vi "add_default_value_on_label.vi"(8 "error in (no error)":errorcluster, 11 "VI Ref In":refnum<vi>) -> (0 "error out":errorcluster, 3 "VI Ref Out":refnum<vi>)   [LabVIEW 2018]
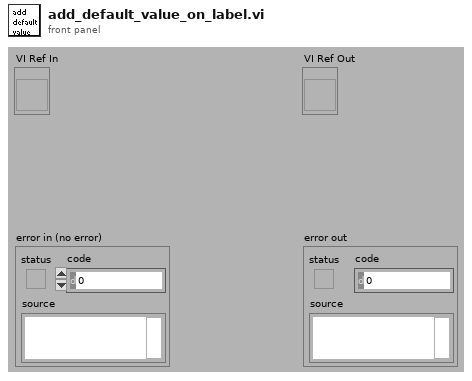
[diagram p1: front panel]
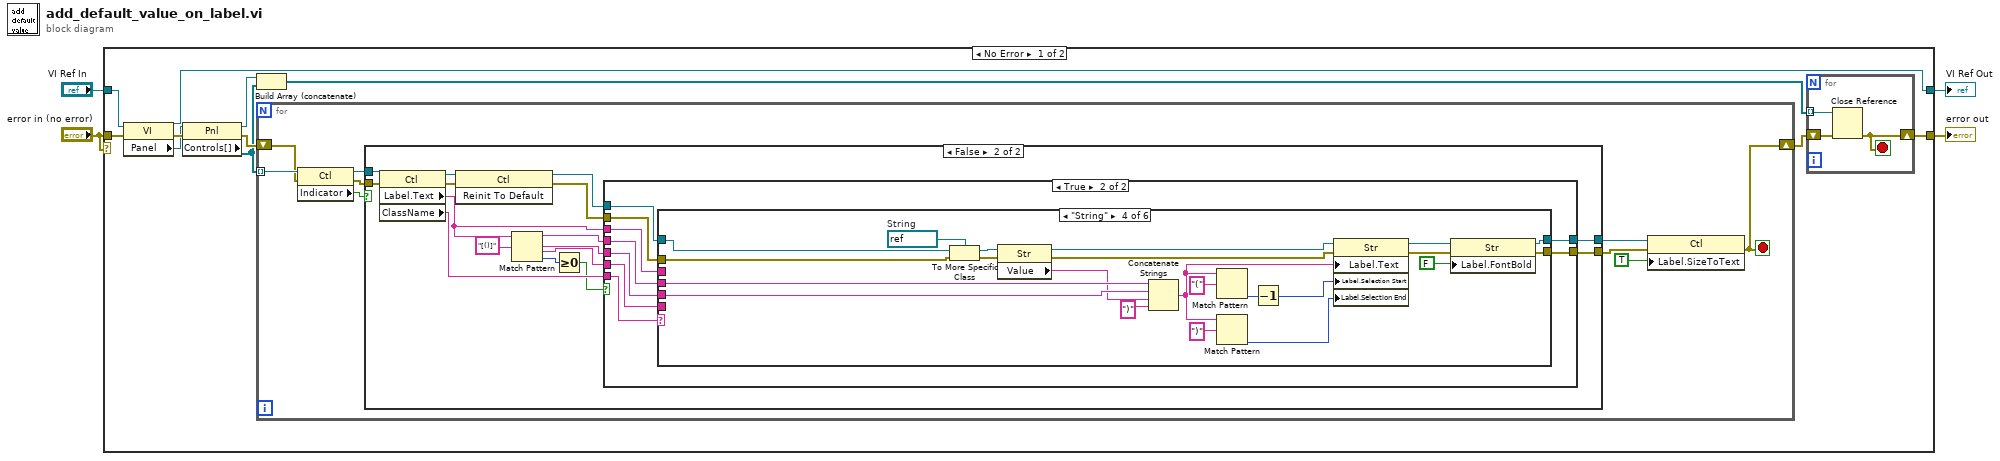
[diagram p0: block diagram]
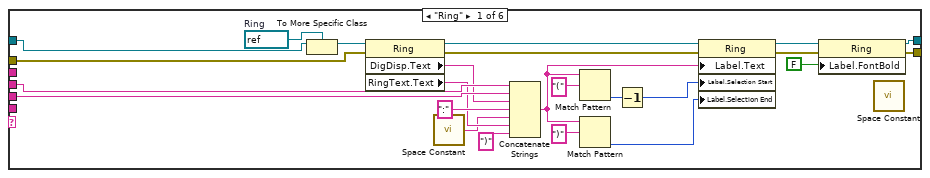
[diagram p4: hidden frame]
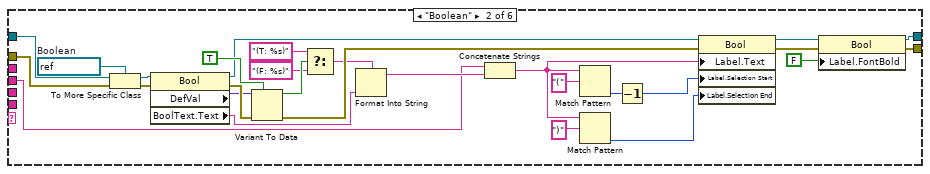
[diagram p5: hidden frame]
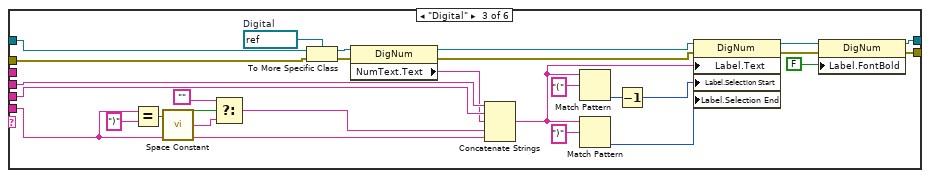
[diagram p6: hidden frame]
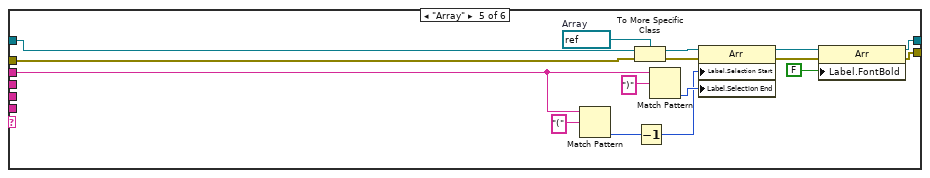
[diagram p7: hidden frame]
diagram:
  n1 = case shown="No Error" "error in (no error)" {
    tunnel: [w9 w177] -> w4
    tunnel: "VI Ref In" -> [w6 w177]
    tunnel: "error in (no error)" -> [w8 w176]
    tunnel: [w7 w176] -> w3
    frame No Error {
      n2 = property class="VI"(reference=w6, error in=w8) -> (reference out=w9:refnum<vi>, error out=w15:errorcluster, "Panel"=w5:refnum<vi>)
      n3 = property class="Pnl"(reference=w5, error in=w15) -> (reference out=w13:refnum<vi>, error out=w14:errorcluster, "Controls[]"=w12:refnum<vi>[])
      n4 = Build Array (concatenate)(w13, w12) -> (w11:refnum<vi>[])
      n5 = for {
        tunnel: w12 -> [w25] mode=indexing
        shift-right: [w19] -> w10
        shift-left: w14 -> [w22]
        stop <- w19 stop-if-true
        n6 = property class="Ctl"(reference=w25, error in=w22) -> (reference out=w23:refnum<vi>, error out=w21:errorcluster, "Indicator"=w24:bool)
        n7 = case shown="False" w24 {
          tunnel: w21 -> [w28 w45]
          tunnel: [w28 w42] -> w20
          tunnel: [w29 w41] -> w27
          tunnel: w23 -> [w29 w40]
          frame True {
          }
          frame False {
            n8 = property class="Ctl"(reference=w40, error in=w45) -> (reference out=w39:refnum<vi>, error out=w38:errorcluster, "Label.Text"=w30:string, "ClassName"=w44:string)
            n9 = invoke class="Ctl" method="Reinit To Default"(reference=w39, error in=w38) -> (reference out=w36:refnum<vi>, error out=w37:errorcluster)  [unwired: 1 in, 1 out]
            n10 = Match Pattern(string=w30, regular expression="[()]") -> (before substring=w33:string, match substring=w32:string, after substring=w31:string, offset past match=w35:i32)  [unwired: 1 out]
            n11 = Greater Or Equal To 0?(x=w35) -> (x >= 0?=w34:bool)
            n12 = case shown="True" w34 {
              tunnel: w37 -> [w47 w56]
              tunnel: w44 -> [_ w54]
              tunnel: w36 -> [w46 w55]
              tunnel: [w47 w53] -> w42
              tunnel: [w46 w52] -> w41
              tunnel: w33 -> [_ w51]
              tunnel: w32 -> [_ w50]
              tunnel: w31 -> [_ w49]
              tunnel: w30 -> [_ w48]
              frame False {
              }
              frame True {
                n13 = case shown="\"String\"" w54 {
                  tunnel: w55 -> [w71 w90 w124 w146 w162 w174]
                  tunnel: w56 -> [w70 w87 w123 w145 w161 w175]
                  tunnel: [w68 w99 w127 w149 w165 w175] -> w53
                  tunnel: [w67 w98 w126 w148 w164 w174] -> w52
                  tunnel: w51 -> [w64 w81 w118 w140 _ _]
                  tunnel: w50 -> [w63 _ w117 w139 _ _]
                  tunnel: w49 -> [_ _ w114 _ _ _]
                  tunnel: w48 -> [_ _ _ _ w158 _]
                  frame "Ring" {
                    w72 = refnum<vi> refnum  # Ring
                    n14 = To More Specific Class(target class=w72, reference=w71) -> (specific class reference=w69:refnum<vi>)  [unwired: 1 in, 1 out]
                    n15 = property class="Ring"(reference=w69, error in=w70) -> (reference out=w66:refnum<vi>, error out=w65:errorcluster, "DigDisp.Text"=w62:string, "RingText.Text"=w60:string)
                    n16 = call <vilib>:"Space Constant.vi"() -> ("String"=w57:string)
                    n17 = Concatenate Strings(w64, w63, w62, ":" ("string"), w57, w60, ")" ("string")) -> (w58:string)
                    n18 = Match Pattern(string=w58, regular expression="(") -> (offset past match=w76:i32)  [unwired: 4 out]
                    n19 = Match Pattern(string=w58, regular expression=")") -> (offset past match=w75:i32)  [unwired: 4 out]
                    n20 = Decrement(x=w76) -> (x-1=w73:i32)
                    n21 = property class="Ring"(reference=w66, error in=w65, "Label.Text"=w58, "Label.Selection Start"=w73, "Label.Selection End"=w75) -> (reference out=w77:refnum<vi>, error out=w78:errorcluster)
                    n22 = property class="Ring"(reference=w77, error in=w78, "Label.FontBold"=FALSE ("Label.Font:Bold")) -> (reference out=w67:refnum<vi>, error out=w68:errorcluster)
                    n23 = call <vilib>:"Space Constant.vi"() -> ()  [unwired: 1 out]
                  }
                  frame "Boolean" {
                    w91 = refnum<vi> refnum  # Boolean
                    n24 = To More Specific Class(target class=w91, reference=w90, error in=w87) -> (specific class reference=w89:refnum<vi>, error out=w88:errorcluster)
                    n25 = property class="Bool"(reference=w89, error in=w88) -> (reference out=w92:refnum<vi>, error out=w97:errorcluster, "DefVal"=w86:variant, "BoolText.Text"=w85:string)
                    n26 = Variant To Data(error in=w97, type=TRUE, Variant=w86) -> (data=w95:bool, error out=w93:errorcluster)
                    n27 = Select(t="(T: %s)" ("string"), s=w95, f="(F: %s)" ("string")) -> (s? t:f=w83:string)
                    n28 = Format Into String(format string=w83, w85) -> (resulting string=w82:string)  [unwired: 2 in, 1 out]
                    n29 = Concatenate Strings(w81, w82) -> (w104:string)
                    n30 = Match Pattern(string=w104, regular expression="(") -> (offset past match=w103:i32)  [unwired: 4 out]
                    n31 = Match Pattern(string=w104, regular expression=")") -> (offset past match=w102:i32)  [unwired: 4 out]
                    n32 = Decrement(x=w103) -> (x-1=w100:i32)
                    n33 = property class="Bool"(reference=w92, error in=w93, "Label.Text"=w104, "Label.Selection Start"=w100, "Label.Selection End"=w102) -> (reference out=w105:refnum<vi>, error out=w106:errorcluster)
                    n34 = property class="Bool"(reference=w105, error in=w106, "Label.FontBold"=FALSE ("Label.Font:Bold")) -> (reference out=w98:refnum<vi>, error out=w99:errorcluster)
                  }
                  frame "Digital" {
                    w125 = refnum<vi> refnum  # Digital
                    n35 = Equal?(x=w114, y=")") -> (x = y?=w112:bool)
                    n36 = call <vilib>:"Space Constant.vi"() -> ("String"=w110:string)
                    n37 = Select(t="", s=w112, f=w110) -> (s? t:f=w109:string)
                    n38 = To More Specific Class(target class=w125, reference=w124, error in=w123) -> (specific class reference=w122:refnum<vi>, error out=w121:errorcluster)
                    n39 = property class="DigNum"(reference=w122, error in=w121) -> (reference out=w120:refnum<vi>, error out=w119:errorcluster, "NumText.Text"=w116:string)
                    n40 = Concatenate Strings(w118, w117, w116, w109, w114) -> (w115:string)
                    n41 = Match Pattern(string=w115, regular expression="(") -> (offset past match=w131:i32)  [unwired: 4 out]
                    n42 = Match Pattern(string=w115, regular expression=")") -> (offset past match=w130:i32)  [unwired: 4 out]
                    n43 = Decrement(x=w131) -> (x-1=w128:i32)
                    n44 = property class="DigNum"(reference=w120, error in=w119, "Label.Text"=w115, "Label.Selection Start"=w128, "Label.Selection End"=w130) -> (reference out=w132:refnum<vi>, error out=w133:errorcluster)
                    n45 = property class="DigNum"(reference=w132, error in=w133, "Label.FontBold"=FALSE ("Label.Font:Bold")) -> (reference out=w126:refnum<vi>, error out=w127:errorcluster)
                  }
                  frame "String" {
                    w147 = refnum<vi> refnum  # String
                    n46 = To More Specific Class(target class=w147, reference=w146, error in=w145) -> (specific class reference=w144:refnum<vi>, error out=w143:errorcluster)
                    n47 = property class="Str"(reference=w144, error in=w143) -> (reference out=w142:refnum<vi>, error out=w141:errorcluster, "Value"=w138:string)
                    n48 = Concatenate Strings(w140, w139, w138, ")" ("string")) -> (w137:string)
                    n49 = Match Pattern(string=w137, regular expression="(") -> (offset past match=w153:i32)  [unwired: 4 out]
                    n50 = Match Pattern(string=w137, regular expression=")") -> (offset past match=w152:i32)  [unwired: 4 out]
                    n51 = Decrement(x=w153) -> (x-1=w150:i32)
                    n52 = property class="Str"(reference=w142, error in=w141, "Label.Text"=w137, "Label.Selection Start"=w150, "Label.Selection End"=w152) -> (reference out=w154:refnum<vi>, error out=w155:errorcluster)
                    n53 = property class="Str"(reference=w154, error in=w155, "Label.FontBold"=FALSE ("Label.Font:Bold")) -> (reference out=w148:refnum<vi>, error out=w149:errorcluster)
                  }
                  frame "Array" {
                    w163 = refnum<vi> refnum  # Array
                    n54 = Match Pattern(string=w158, regular expression="(") -> (offset past match=w169:i32)  [unwired: 4 out]
                    n55 = To More Specific Class(target class=w163, reference=w162, error in=w161) -> (specific class reference=w160:refnum<vi>, error out=w159:errorcluster)
                    n56 = Decrement(x=w169) -> (x-1=w166:i32)
                    n57 = Match Pattern(string=w158, regular expression=")") -> (offset past match=w168:i32)  [unwired: 4 out]
                    n58 = property class="Arr"(reference=w160, error in=w159, "Label.Selection Start"=w166, "Label.Selection End"=w168) -> (reference out=w170:refnum<vi>, error out=w171:errorcluster)
                    n59 = property class="Arr"(reference=w170, error in=w171, "Label.FontBold"=FALSE ("Label.Font:Bold")) -> (reference out=w164:refnum<vi>, error out=w165:errorcluster)
                  }
                  frame Default {
                  }
                }
              }
            }
          }
        }
        n60 = property class="Ctl"(reference=w27, error in=w20, "Label.SizeToText"=TRUE ("Label.Size to Text?")) -> (error out=w19:errorcluster)  [unwired: 1 out]
      }
      n61 = for {
        tunnel: w11 -> [w18] mode=indexing
        shift-right: [w16] -> w7
        shift-left: w10 -> [w17]
        stop <- w16 stop-if-true
        n62 = Close Reference(reference=w18, error in (no error)=w17) -> (error out=w16:errorcluster)
      }
    }
    frame Error {
    }
  }
  "VI Ref Out" <- w4
  "error out" <- w3
